vi "Shutdown HW.vi"(8 "error in (no error)":errorcluster, 11 "Servo in":refnum<class "Servo.lvclass">) -> (0 "error out":errorcluster, 3 "Servo out":refnum<class "Servo.lvclass">)   [LabVIEW 2020, in "Servo.lvclass"]
uses:
  Servo.lvclass
  Actuator.lvclass
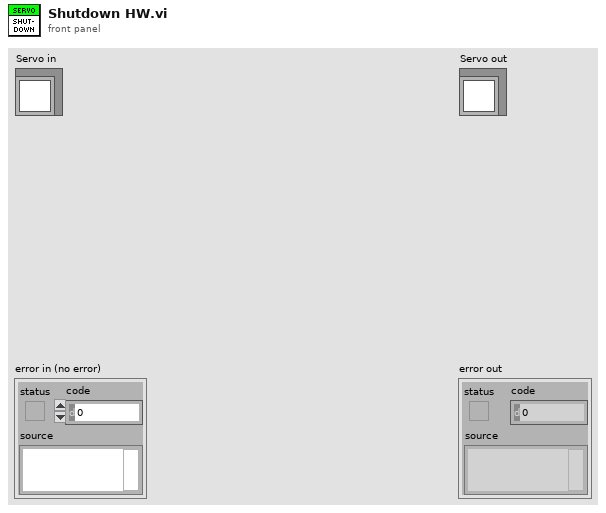
[diagram p1: front panel]
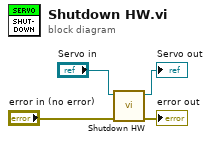
[diagram p0: block diagram]
diagram:
  n1 = call-parent "Shutdown HW.vi"("error in (no error)"="error in (no error)", "Actuator in"="Servo in") -> ("error out"=→"error out":errorcluster, "Actuator out"=→"Servo out":refnum<class "Servo.lvclass">)  [unwired: 8 in]
